vi "FindKeyTiming.vi"() -> ()   [LabVIEW 2020]
uses:
  controls/Gameboard Data.ctl
  controls/Player.ctl
panel:
  in  "No. of iterations":i32=100
  out "BuildDecisionTree (s)":dbl
  out "BuildDecisionTree_alt (s)":dbl
  # "Times BuildDecisionTree.vi with simpler FindTreeKey.vi that potentialy repeatedly asks for the same key \nand an alternative version with FindTreeKey_alt.vi that eliminates duplicates via creating a map and asking for elements from it"
  # "100 iteration of each takes some time \nbut not too much"
  # "my results were 0.12166 s for original\nand 0.16079 s for alt. The first version stays"
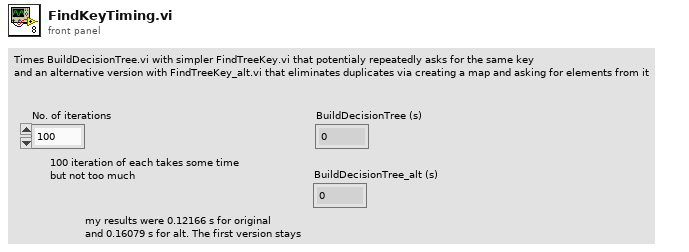
[diagram p1: front panel]
types:
  T1 = typedef "Player.ctl" = enum16{"None", "Player 1", "Player 2"}
  T2 = typedef "Gameboard Data.ctl" = enum16{"None", "Player 1", "Player 2"}[]
  T3 = typedef "DecisionTree.ctl" = map{T2, T4}
  T4 = typedef "DecisionTreeRecord.ctl" = cluster{"Status":T1, "GoodMoves":i8[], "MehMoves":i8[], "BadMoves":i8[]}
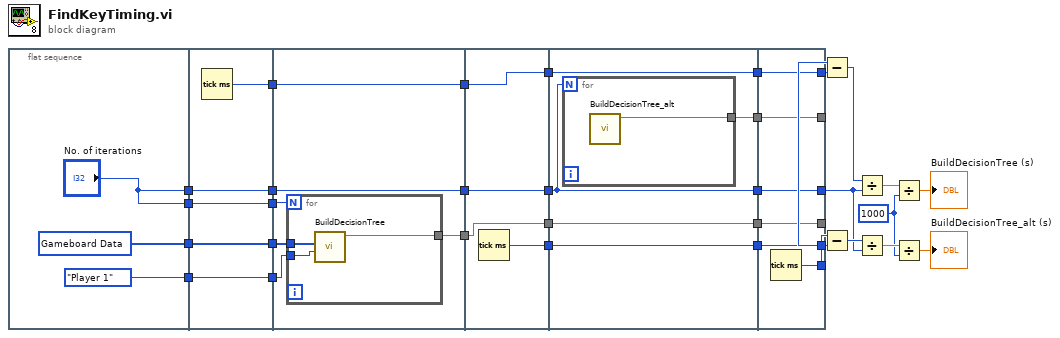
[diagram p0: block diagram]
diagram:
  w5 = 1000
  n1 = flat-sequence {
    tunnel: [Player."Player 1" ("Current Player")] -> w22
    tunnel: [w34] -> w20
    tunnel: ["No. of iterations"] -> w14
    tunnel: ["No. of iterations"] -> w10
    tunnel: [w40] -> w24
    tunnel: [w39] -> w23
    tunnel: w22 -> [w39]
    tunnel: [w38] -> w21
    tunnel: w20 -> [w38]
    tunnel: [w37] -> w15
    tunnel: w14 -> [w37]
    tunnel: [w36] -> w11
    tunnel: w10 -> [w36]
    tunnel: [w46] -> w25
    tunnel: w24 -> [w46]
    tunnel: w23 -> [w45]
    tunnel: w21 -> [w44]
    tunnel: [w43] -> w17
    tunnel: w15 -> [w42]
    tunnel: [w41] -> w12
    tunnel: w11 -> [w41]
    tunnel: [w53] -> w31
    tunnel: [w52] -> w26
    tunnel: w25 -> [w52]
    tunnel: [w51] -> w18
    tunnel: w17 -> [w51]
    tunnel: [w50] -> w13
    tunnel: w12 -> [w50]
    tunnel: w31 -> [w58]
    tunnel: [w58] -> w30
    tunnel: [w57] -> w27
    tunnel: w26 -> [w57]
    tunnel: [w56] -> w19
    tunnel: w18 -> [w56]
    tunnel: [w55] -> w16
    tunnel: w13 -> [w54]
    tunnel: [w54] -> w1
    tunnel: [w65] -> w32
    tunnel: w30 -> [w64]
    tunnel: [w64] -> w29
    tunnel: [w63] -> w28
    tunnel: w27 -> [w63]
    tunnel: [w62] -> _
    tunnel: w19 -> [w62]
    tunnel: [w61] -> _
    tunnel: w16 -> [w61]
    tunnel: [w60] -> w2
    tunnel: w1 -> [w60]
    frame #0 {
      w34 = T2 [enum."None", enum."None", enum."None", enum."None", enum."None", enum."None", enum."None", enum."None", enum."None"] items=["None", "Player 1", "Player 2"] ("Gameboard")
    }
    frame #1 {
      n2 = Tick Count (ms)() -> (millisecond timer value=w40:u32)
    }
    frame #2 {
      n3 = for {
        N: w42 -> [_]
        tunnel: w45 -> [w49]
        tunnel: w44 -> [w48]
        tunnel: [w47] -> w43
        n4 = call "BuildDecisionTree.vi"("Current Player"=w49, "Gameboard"=w48) -> ("DecisionTree Out"=w47:T3)  [unwired: 7 in, 2 out]
      }
    }
    frame #3 {
      n5 = Tick Count (ms)() -> (millisecond timer value=w53:u32)
    }
    frame #4 {
      n6 = for {
        N: w54 -> [_]
        tunnel: [w59] -> w55
        n7 = call "BuildDecisionTree_alt.vi"() -> ("DecisionTree Out"=w59:T3)  [unwired: 9 in, 2 out]
      }
    }
    frame #5 {
      n8 = Tick Count (ms)() -> (millisecond timer value=w65:u32)
    }
  }
  n9 = Subtract(x=w29, y=w28) -> (x-y=w8:u32)
  n10 = Subtract(x=w32, y=w29) -> (x-y=w9:u32)
  n11 = Divide(x=w8, y=w2) -> (x/y=w6:dbl)
  n12 = Divide(x=w9, y=w2) -> (x/y=w7:dbl)
  n13 = Divide(x=w6, y=w5) -> (x/y=→"BuildDecisionTree (s)":dbl)
  n14 = Divide(x=w7, y=w5) -> (x/y=→"BuildDecisionTree_alt (s)":dbl)
